vi "Get Pulse Width.vi"(8 "error in (no error)":errorcluster, 11 "Servo in":refnum<class "Servo.lvclass">) -> (0 "error out":errorcluster, 2 "pulse width (micro-sec)":dbl, 3 "Servo out":refnum<class "Servo.lvclass">)   [LabVIEW 2020, in "Servo.lvclass"]
uses:
  Servo.lvclass
  Servo.lvclass/Servo.ctl
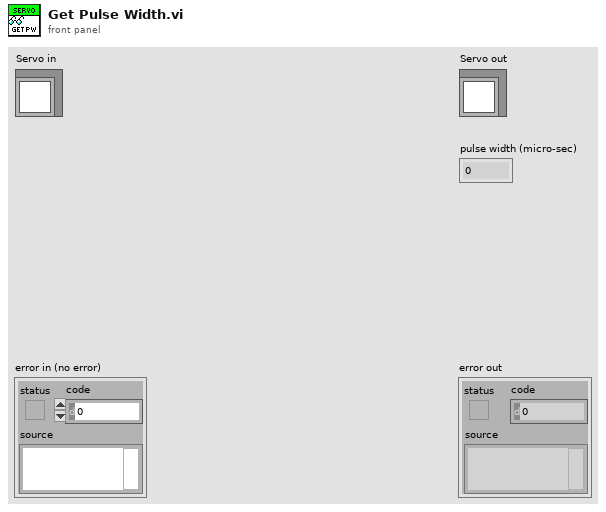
[diagram p1: front panel]
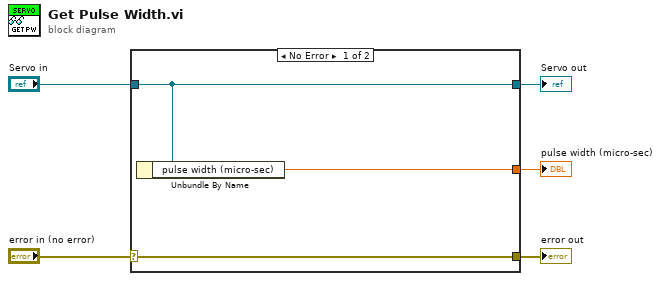
[diagram p0: block diagram]
diagram:
  n1 = case shown="No Error" "error in (no error)" {
    selector: "error in (no error)" -> [w8 w9]
    tunnel: [w8 w9] -> w4
    tunnel: [w7 w10] -> w2
    tunnel: "Servo in" -> [w7 w10]
    tunnel: [w6 _] -> w1
    frame No Error {
      n2 = Unbundle By Name(w7) -> ("pulse width (micro-sec)"=w6:dbl)
    }
    frame Error {
    }
  }
  "error out" <- w4
  "Servo out" <- w2
  "pulse width (micro-sec)" <- w1
